vi "setLevel.vi"(8 "error in (no error)":errorcluster, 10 "Level":dbl, 11 "Tank in":refnum<class "Tank.lvclass">) -> (0 "error out":errorcluster, 3 "Tank out":refnum<class "Tank.lvclass">)   [LabVIEW 2017, in "Tank.lvclass"]
uses:
  Tank.lvclass
  Tank.lvclass/Tank.ctl
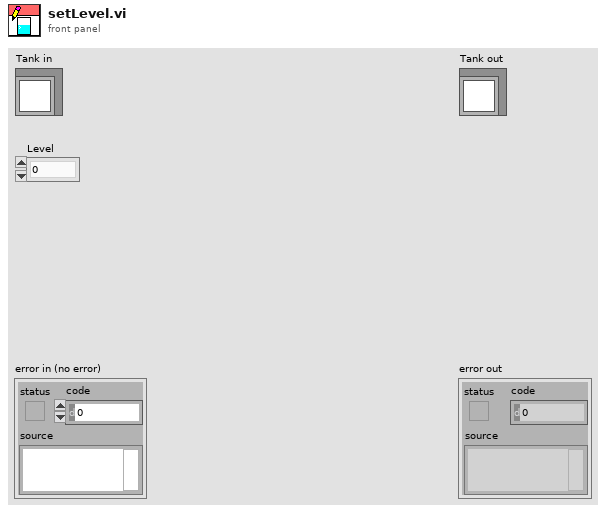
[diagram p1: front panel]
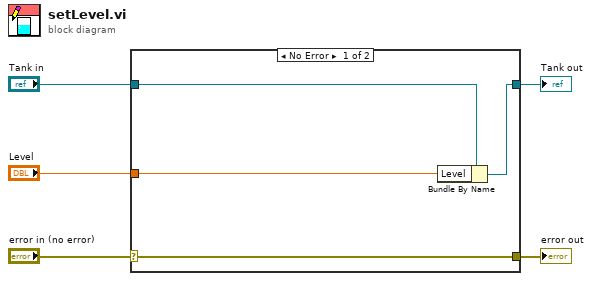
[diagram p0: block diagram]
diagram:
  n1 = case shown="No Error" "error in (no error)" {
    selector: "error in (no error)" -> [w9 w10]
    tunnel: [w9 w10] -> w4
    tunnel: [w7 w11] -> w2
    tunnel: "Tank in" -> [w8 w11]
    tunnel: "Level" -> [w6 _]
    frame No Error {
      n2 = Bundle By Name(cluster=w8, "Level"=w6) -> (w7:refnum<class "Tank.lvclass">)
    }
    frame Error {
    }
  }
  "error out" <- w4
  "Tank out" <- w2
